vi "uTransport_uActor_SendMsg.vi"(8 "error in (no error)":errorcluster, 10 "Msg":refnum<class "uMsg.lvclass">, 11 "uTransport_uActor in":refnum<class "uTransport_uActor.lvclass">) -> (0 "error out":errorcluster)   [LabVIEW 2023, in "uLib.lvlib" / "uTransport_uActor.lvclass"]
doc: "Use instead of the interface's 'SendMsg' method when high speed streaming is a priority. This is inlined to optimize for performance."
uses:
  uTransport_uActor.lvclass
  uMsg/uMsg/uMsg.lvclass
  uTransport_uActor.lvclass/uTransport_uActor.ctl
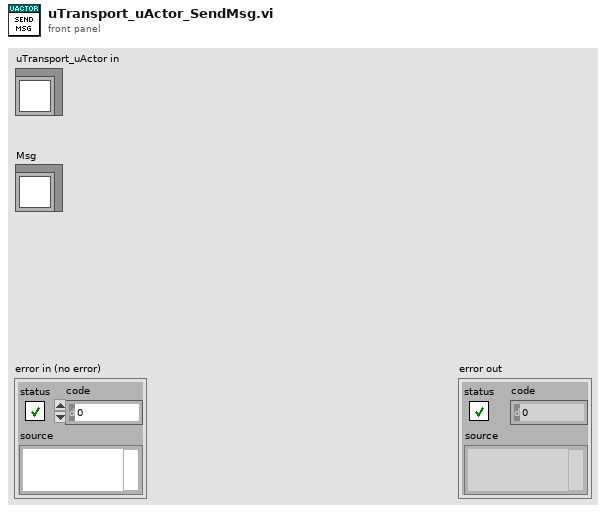
[diagram p1: front panel]
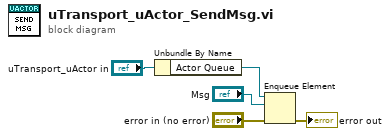
[diagram p0: block diagram]
diagram:
  n1 = Unbundle By Name("uTransport_uActor in") -> ("Actor Queue"=w2:refnum<queue>)
  n2 = Enqueue Element(queue=w2, element="Msg", error in (no error)="error in (no error)") -> (error out=→"error out":errorcluster)  [unwired: 1 in, 2 out]
